vi "Save image.vi"(7 "image number":i32, 8 "error in":errorcluster, 10 "image data":u8[](array[numeric]), 11 "folder (dialog)":path) -> (0 "error out":errorcluster, 2 "image path":path)   [LabVIEW 2013]
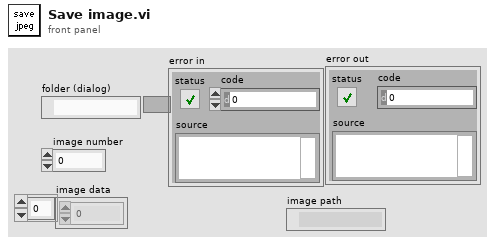
[diagram p1: front panel]
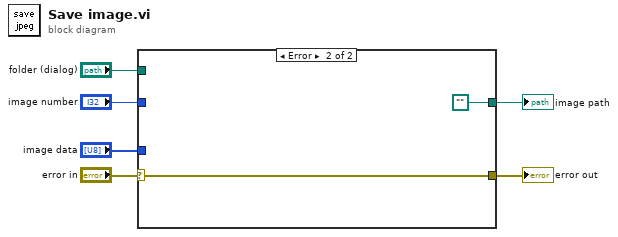
[diagram p0: block diagram]
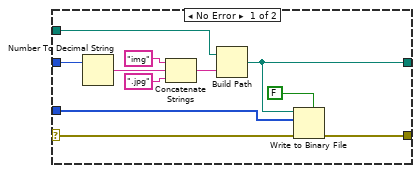
[diagram p2: hidden frame]
diagram:
  n1 = case shown="Error" "error in" {
    selector: "error in" -> [w8 w19]
    tunnel: "image data" -> [w17 _]
    tunnel: "image number" -> [w11 _]
    tunnel: "folder (dialog)" -> [w10 _]
    tunnel: [w9 w19] -> w3
    tunnel: [w7 path ""] -> w1
    frame No Error {
      n2 = Number To Decimal String(number=w11) -> (decimal integer string=w13:string)  [unwired: 1 in]
      n3 = Concatenate Strings("img", w13, ".jpg" ("string")) -> (w14:string)
      n4 = Build Path(base path=w10, name or relative path=w14) -> (appended path=w7:path)
      n5 = Write to Binary File(file (use dialog)=w7, data=w17, error in=w8, 5:FALSE ("prepend array or string size? (T)")) -> (error out=w9:errorcluster)  [unwired: 2 in, 2 out]
    }
    frame Error {
    }
  }
  "error out" <- w3
  "image path" <- w1
